vi "FolloWin.vi"() -> ()   [LabVIEW 2023, in "FolloWin.lvclass"]
doc: "This is the actual window that follows the cursor, it is controlled externally through the class methods."
uses:
  FolloWin.lvclass
  <vilib>/Utility/miscctls.llb/LVRectTypeDef.ctl
  <vilib>/Utility/inputDevices.llb/mouseAcquire.vi
  <vilib>/Utility/inputDevices.llb/closeMouse.vi
panel:
  out "String":string
  out "Comment":string="Thid is the FolloWin window that follows the mouse cursor. \nthe only part that the user should sees of this front panel is the green rectangle (positioned at 0,0)\nDO NOT ADD ANY DECORATIONS TO THIS FRONT PANEL\nThe ONLY decoration should be the green box\n(this is why this comment is a string and not a label which is a decoration)"
  in  "ms per cycle":u32=16
  in  "Transparency":u8=50
  in  "Box bound":T1
  in  "Hidden?":bool=TRUE
  in  "Height":i32
  in  "Width":i32
  in  "Y offset":i32
  in  "X offset":i32
  in  "Stop?":bool=TRUE
  out "2D Picture":picture
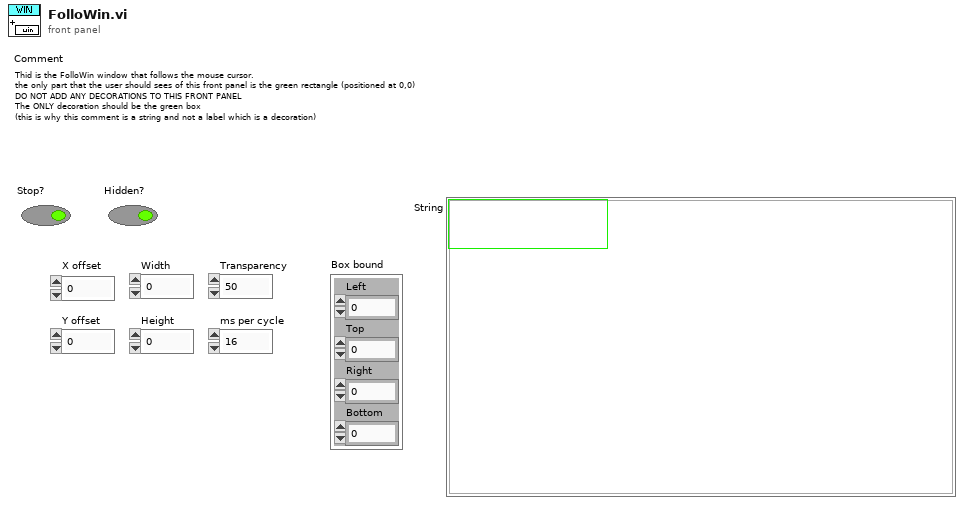
[diagram p1: front panel]
types:
  T1 = typedef "LVRectTypeDef.ctl" = cluster{"Left":i16, "Top":i16, "Right":i16, "Bottom":i16}
  T2 = enum32{"Invalid", "Standard", "Closed", "Hidden", "Minimized", "Maximized"}
  T3 = enum16{"Biggest", "Rightmost", "Leftmost", "Topmost", "Bottommost"}
  T4 = cluster{"Horizontal":i32, "Vertical":i32, "Scrolling":i32}
  T5 = cluster{"button 1":bool, "button 2":bool, "button 3":bool, "button 4":bool}
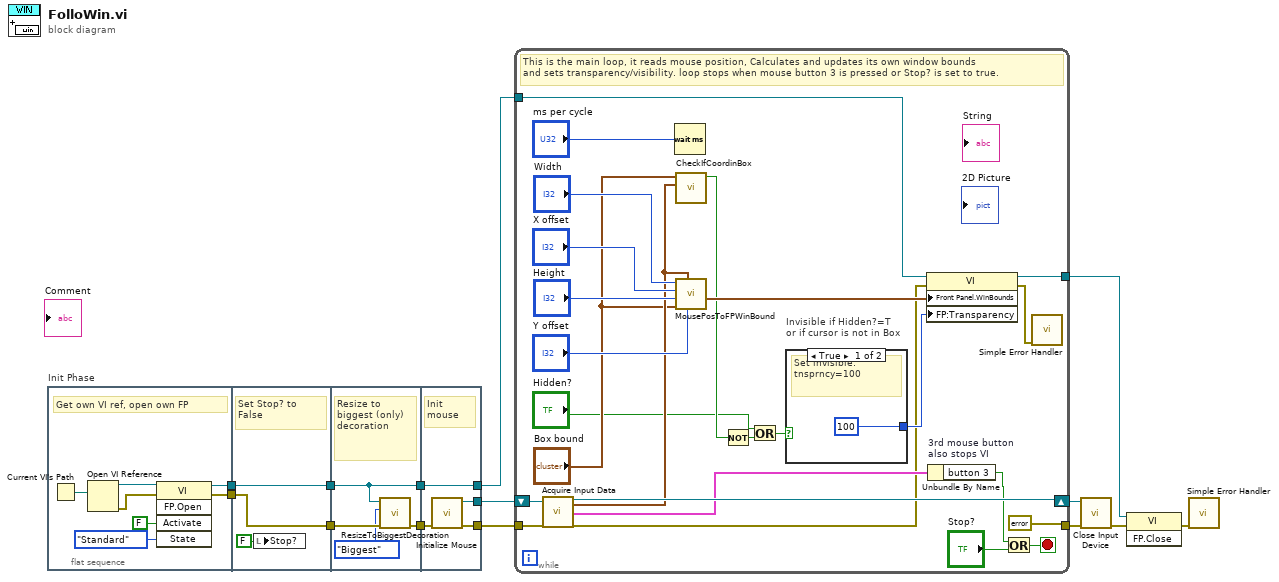
[diagram p0: block diagram]
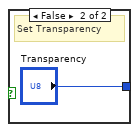
[diagram p2: hidden frame]
diagram:
  n1 = flat-sequence "Init Phase" {
    tunnel: [w15] -> w8
    tunnel: [w16] -> w7
    tunnel: [w24] -> w10
    tunnel: [w23] -> w9
    tunnel: w8 -> [w24]
    tunnel: w7 -> [w23]
    tunnel: w10 -> [w28]
    tunnel: w9 -> [w26]
    tunnel: [w27] -> w4
    tunnel: [w26] -> w3
    tunnel: [w32] -> w6
    tunnel: w4 -> [w31]
    tunnel: w3 -> [w32]
    tunnel: [w30] -> w2
    tunnel: [w29] -> w1
    frame #0 {
      # "Get own VI ref, open own FP"
      n2 = Current VI's Path() -> (path=w19:path)
      n3 = Open VI Reference(vi path=w19) -> (vi reference=w20:refnum<vi>, error out=w21:errorcluster)  [unwired: 5 in]
      n4 = invoke on="Invoke Node" class="VI" method="FP.Open"(reference=w20, error in=w21, "Activate"=FALSE ("Activate?"), "State"=T2."Standard") -> (reference out=w16:refnum<vi>, error out=w15:errorcluster)  [unwired: 1 in, 3 out]
    }
    frame #1 {
      # "Set Stop? to False"
      n5 = local write "Stop?"(FALSE ("Boolean")) -> ()
    }
    frame #2 {
      # "Resize to biggest (only) decoration"
      n6 = call "ResizeToBiggestDecoration.vi"("error in (no error)"=w28, "Resize By"=T3."Biggest", "VI in"=w26) -> ("error out"=w27:errorcluster)  [unwired: 8 in]
    }
    frame #3 {
      # "Init mouse"
      n7 = call <vilib>:"Initialize Mouse.vi"("error in (no error)"=w31) -> ("error out"=w30:errorcluster, "device ID"=w29:refnum<k1>)  [unwired: 9 in]
    }
  }
  n8 = while {
    tunnel: w2 -> [w56]
    tunnel: [errorcluster {"status"=FALSE, "code"=0, "source"=""} ("error out")] -> w14
    tunnel: w6 -> [w54]
    tunnel: [w49] -> w11
    shift-right: [w55] -> w13
    shift-left: w1 -> [w57]
    stop <- w50 stop-if-true
    # "This is the main loop, it reads mouse position, Calculates and updates its own window bounds \nand sets transparency/visibility. loop stops when mouse button 3 is pressed or Stop? is set to true."
    n9 = call-poly <vilib>:"Acquire Input Data.vi"("device ID"=w57, "error in (no error)"=w56) -> ("device ID"=w55:refnum<k1>, "axis info"=w44:T4, "button info"=w52:T5, "error out"=w35:errorcluster)  [unwired: 14 in]
    n10 = Wait (ms)(milliseconds to wait="ms per cycle") -> ()  [unwired: 1 out]
    n11 = call "CheckIfCoordinBox.vi"("axis info"=w44, "Box bounds"="Box bound") -> ("In Box"=w41:bool)  [unwired: 9 in]
    n12 = call "MousePosToFPWinBound.vi"("Y offset"="Y offset", "axis info"=w44, "Active Box"="Box bound", "Height"="Height", "X offset"="X offset", "Width"="Width") -> ("Output Bounds"=w53:T1)  [unwired: 5 in]
    n13 = Not(x=w41) -> (.not. x?=w39:bool)
    n14 = Or(x="Hidden?", y=w39) -> (x .or. y?=w37:bool)
    n15 = case "Invisible if Hidden?=T \nor if cursor is not in Box" shown="True" w37 {
      tunnel: [u8 100 ("Front Panel Window:Transparency") "Transparency"] -> w40
      frame True {
        # "Set invisible: tnsprncy=100"
      }
      frame False {
        # "Set Transparency"
      }
    }
    n16 = property on="Property Node" class="VI"(reference=w54, error in=w35, "Front Panel.WinBounds"=w53, "FP:Transparency"=w40) -> (reference out=w49:refnum<vi>, error out=w34:errorcluster)
    n17 = Unbundle By Name "3rd mouse button \nalso stops VI"(w52) -> ("button 3"=w43:bool)
    n18 = Or(x=w43, y="Stop?") -> (x .or. y?=w50:bool)
    n19 = call <vilib>:"Simple Error Handler.vi"("error in (no error)"=w34) -> ()  [unwired: 4 in, 5 out]
  }
  n20 = call-poly <vilib>:"Close Input Device.vi"("error in (no error)"=w14, "device ID"=w13) -> ("error out"=w12:errorcluster)  [unwired: 8 in]
  n21 = invoke on="Invoke Node" class="VI" method="FP.Close"(reference=w11, error in=w12) -> (error out=w5:errorcluster)  [unwired: 1 in, 2 out]
  n22 = call <vilib>:"Simple Error Handler.vi"("error in (no error)"=w5) -> ()  [unwired: 4 in, 5 out]
